vi "bin2float32.vi"(9 "Binary":bool[](array[boolean])) -> (1 "Result":ext)   [LabVIEW 2020]
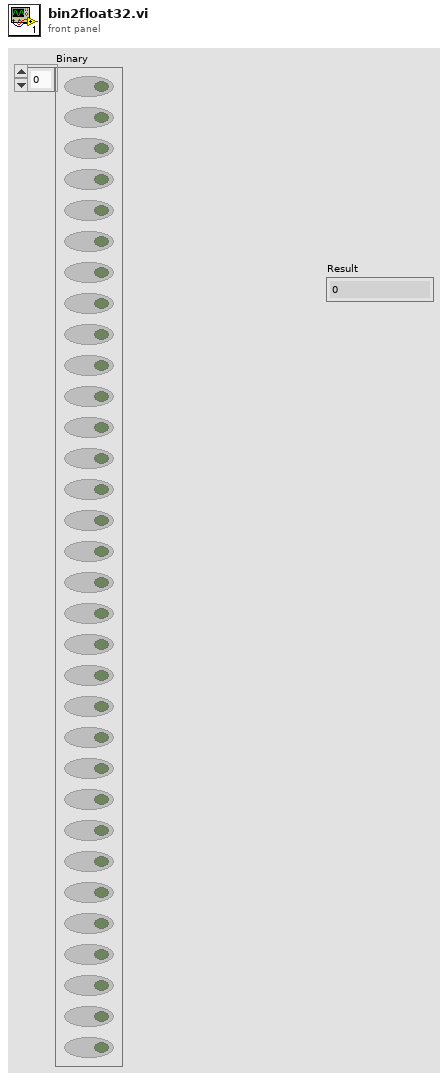
[diagram p1: front panel]
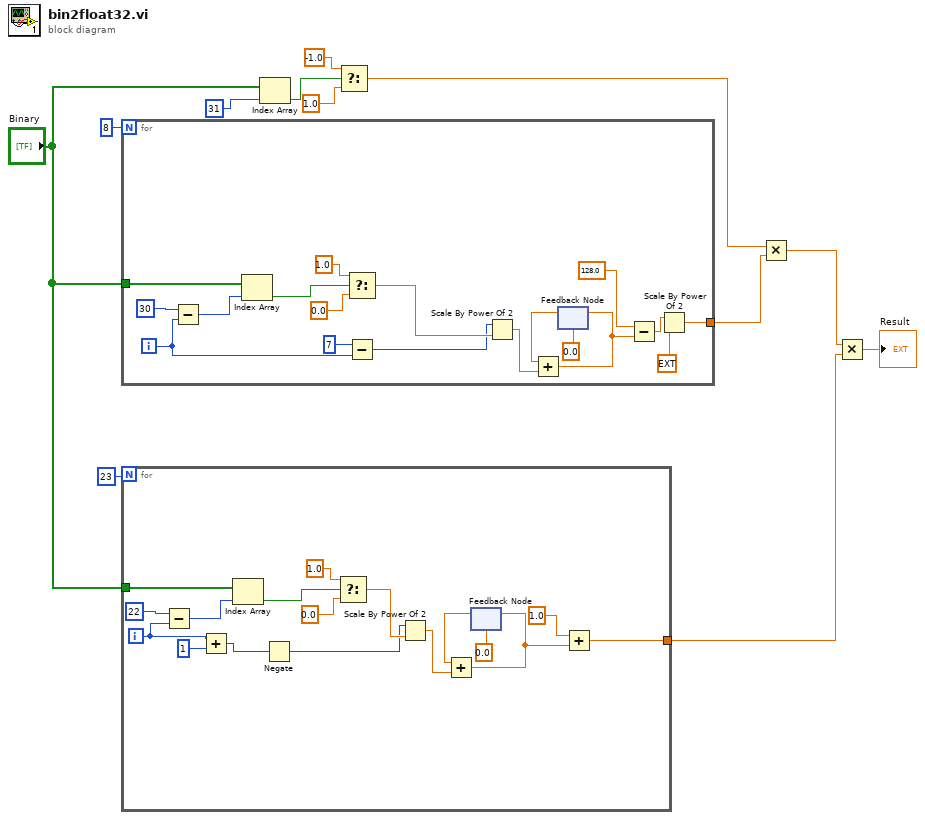
[diagram p0: block diagram]
diagram:
  n1 = for {
    N: 8 -> [_]
    tunnel: "Binary" -> [w27]
    tunnel: [w13] -> w5
    i -> [w19]
    n2 = Subtract(x=30, y=w19) -> (x-y=w21:i32)
    n3 = Index Array(array=w27, index=w21) -> (element=w24:bool)
    n4 = Select(t=1.0, s=w24, f=0.0) -> (s? t:f=w23:dbl)
    n5 = Subtract(x=7, y=w19) -> (x-y=w20:i32)
    n6 = Scale By Power Of 2(n=w20, x=w23) -> (x*2^n=w28:dbl)
    n7 = feedback #1(0.0) -> (w30:dbl)
    n8 = Add(x=w30, y=w28) -> (x+y=w16:dbl)
    n9 = feedback-in #1(w16) -> ()
    n10 = Subtract(x=128.0, y=w16) -> (x-y=w15:dbl)
    n11 = Scale By Power Of 2(n=w15, x=ext 1.0) -> (x*2^n=w13:ext)
  }
  n12 = for {
    N: 23 -> [_]
    tunnel: "Binary" -> [w39]
    tunnel: [w31] -> w2
    i -> [w34]
    n13 = Subtract(x=22, y=w34) -> (x-y=w41:i32)
    n14 = Add(x=w34, y=1) -> (x+y=w32:i32)
    n15 = Index Array(array=w39, index=w41) -> (element=w40:bool)
    n16 = Negate(x=w32) -> (-x=w37:i32)
    n17 = Select(t=1.0, s=w40, f=0.0) -> (s? t:f=w42:dbl)
    n18 = Scale By Power Of 2(n=w37, x=w42) -> (x*2^n=w45:dbl)
    n19 = feedback #2(0.0) -> (w47:dbl)
    n20 = Add(x=w47, y=w45) -> (x+y=w36:dbl)
    n21 = feedback-in #2(w36) -> ()
    n22 = Add(x=1.0, y=w36) -> (x+y=w31:dbl)
  }
  n23 = Index Array(array="Binary", index=31) -> (element=w10:bool)
  n24 = Select(t=-1.0, s=w10, f=1.0) -> (s? t:f=w4:dbl)
  n25 = Multiply(x=w4, y=w5) -> (x*y=w3:ext)
  n26 = Multiply(x=w3, y=w2) -> (x*y=→"Result":ext)
